vi "WS_RS485ETH_only_read.vi"(8 "error in":errorcluster, 11 "conn_id_in":refnum<k5>) -> (0 "error out":errorcluster, 2 "response":string, 3 "conn_id_out":refnum<k5>, 4 "status":bool)   [LabVIEW 2019]
panel:
  in  "timeout ms":i32=1000
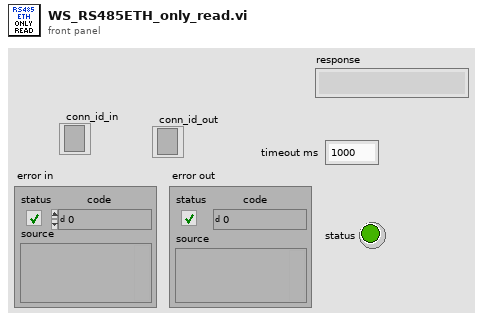
[diagram p1: front panel]
types:
  T1 = enum16{"Standard", "Buffered", "CRLF", "Immediate"}
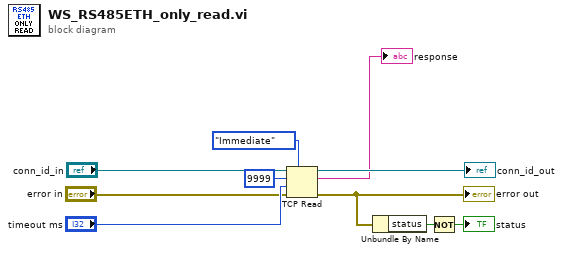
[diagram p0: block diagram]
diagram:
  n1 = TCP Read(connection ID="conn_id_in", bytes to read=9999, error in (no error)="error in", 7:T1."Immediate" ("mode (standard)"), 9:"timeout ms") -> (connection ID out=→"conn_id_out":refnum<k5>, data out=→"response":string, error out=w8:errorcluster)
  "error out" <- w8
  n2 = Unbundle By Name(w8) -> ("status"=w7:bool)
  n3 = Not(x=w7) -> (.not. x?=→"status":bool)
